vi "Get Scanner.vi"(8 "error in (no error)":errorcluster, 11 "Spectrometer Digikröm and PEM in":refnum<class "Spectrometer Digikröm and PEM.lvclass">) -> (0 "error out":errorcluster, 2 "Default Scanner out":refnum<class "Scanner.lvclass">)   [LabVIEW 2017, in "Spectrometer Digikröm and PEM.lvclass"]
doc: "(Dynamic) Returns the default Scanner object that scans over this Scannable. (Note that a Scannable may have multiple Scanners associated with it.) A Scanner is an analogue to an Iterator class in other languages."
uses:
  Scanners/Scanner/Scanner.lvclass
  Utility Classes/Scannable/Scannable.lvclass
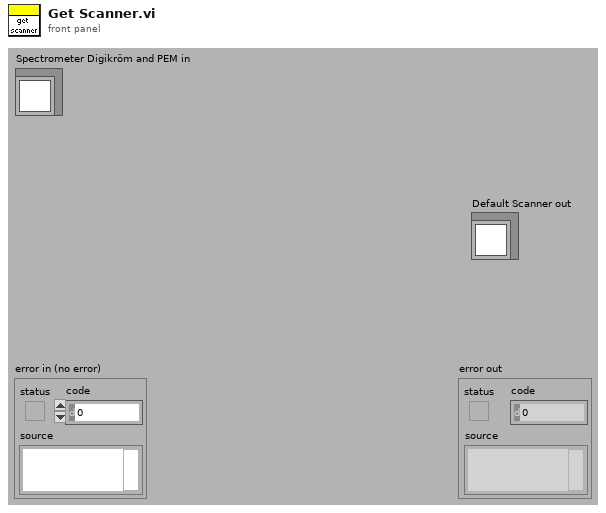
[diagram p1: front panel]
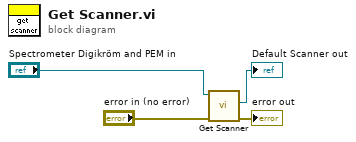
[diagram p0: block diagram]
diagram:
  n1 = call-parent "Get Scanner.vi"("error in (no error)"="error in (no error)", "Scannable in"="Spectrometer Digikröm and PEM in") -> ("error out"=→"error out":errorcluster, "Default Scanner out"=→"Default Scanner out":refnum<class "Scanner.lvclass">)  [unwired: 8 in]
